vi "Calculate F(x) improved performance.vi"() -> (2 "val1":dbl, 3 "f(x)":dbl)   [LabVIEW 2020]
panel:
  out "Waveform Graph 2":dbl[](graph)
  out "Waveform Graph":dbl[](graph)
  out "Output Array":dbl[][](array[numeric])
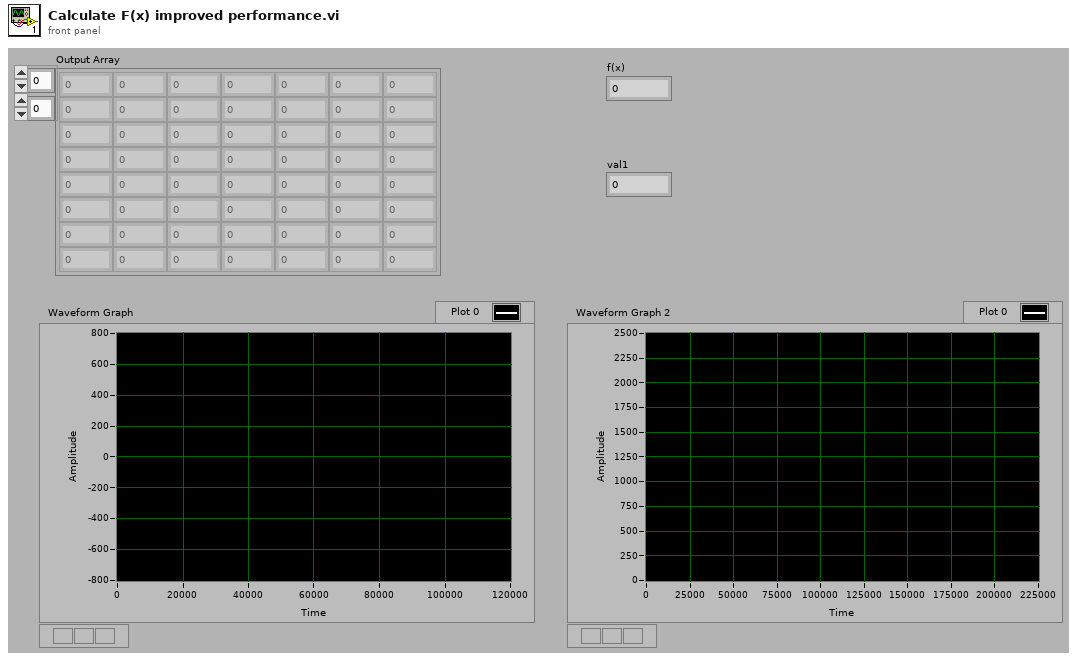
[diagram p1: front panel]
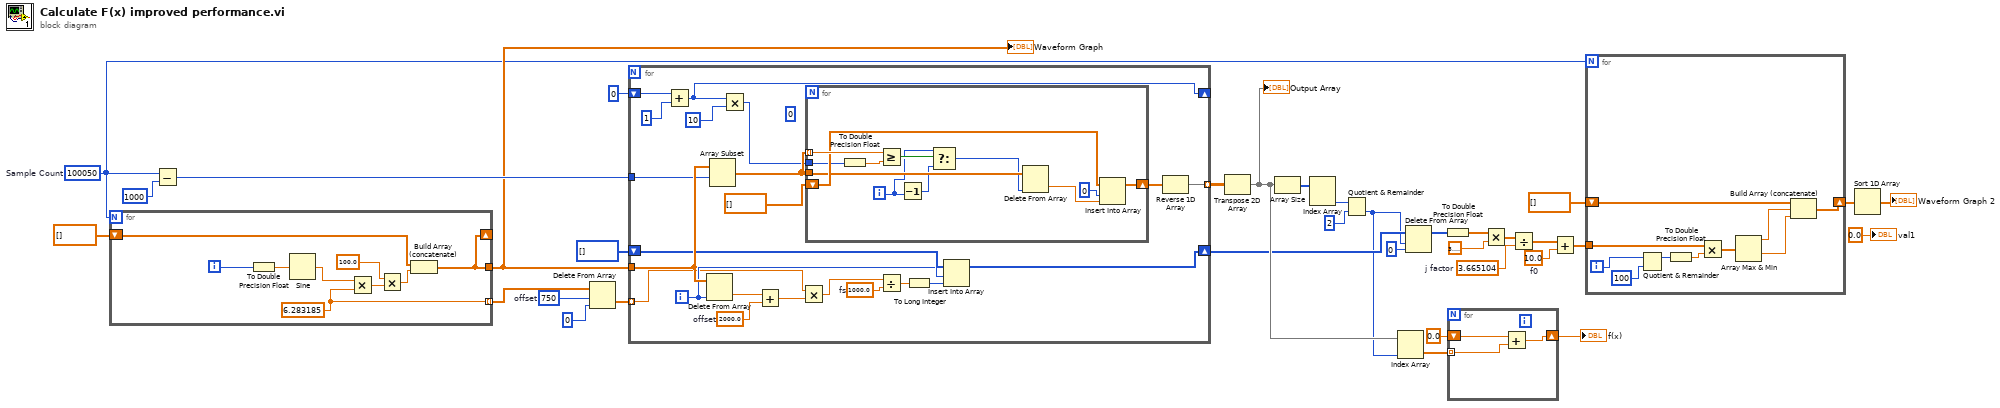
[diagram p0: block diagram]
diagram:
  w10 = 10.0  # f0
  w9 = 3.665104  # j factor
  w17 = 100050  # Sample Count
  w19 = 750  # offset
  n1 = for {
    N: w17 -> [_]
    tunnel: [w38] -> w31 mode=indexing
    tunnel: [w41] -> w18
    shift-right: [w41] -> _
    shift-left: dbl[] [] -> [w40]
    i -> [w42]
    w38 = 6.283185
    n2 = To Double Precision Float(number=w42) -> (double precision float=w43:dbl)
    n3 = Sine(x=w43) -> (sin(x)=w39:dbl)
    n4 = Multiply(x=w39, y=w38) -> (x*y=w37:dbl)
    n5 = Multiply(x=100.0, y=w37) -> (x*y=w35:dbl)
    n6 = Build Array (concatenate)(w40, w35) -> (w41:dbl[])
  }
  "Waveform Graph" <- w18
  n7 = Subtract(x=w17, y=1000) -> (x-y=w22:i32)
  n8 = Delete From Array(array=w31, length=w19, index=0) -> (deleted portion=w20:dbl[])  [unwired: 1 out]
  n9 = for {
    tunnel: w18 -> [w56]
    tunnel: w22 -> [w48]
    tunnel: [w62] -> w34 mode=indexing
    shift-right: [w59] -> _
    shift-left: 0 -> [w60]
    shift-right: [w54] -> w8
    shift-left: i32[] [] -> [w55]
    tunnel: w20 -> [w52] mode=indexing
    i -> [w53]
    w44 = 1000.0  # fs
    w47 = 2000.0  # offset
    (unwired) 0
    n10 = Add(x=w60, y=1) -> (x+y=w59:i32)
    n11 = Delete From Array(array=w56, index=w53) -> (deleted portion=w51:dbl)  [unwired: 1 in, 1 out]
    n12 = Array Subset(array=w56, index=w48) -> (w65:dbl[])  [unwired: 1 in]
    n13 = Multiply(x=w59, y=10) -> (x*y=w57:i32)
    n14 = Add(x=w51, y=w47) -> (x+y=w46:dbl)
    n15 = Multiply(x=w52, y=w46) -> (x*y=w45:dbl)
    n16 = for {
      tunnel: w65 -> [w77] mode=indexing
      tunnel: w65 -> [w74]
      shift-right: [w75] -> w63
      shift-left: dbl[] [] ("array") -> [w76]
      tunnel: w57 -> [w71]
      i -> [w67]
      n17 = To Double Precision Float(number=w71) -> (double precision float=w70:dbl)
      n18 = Greater Or Equal?(x=w77, y=w70) -> (x >= y?=w69:bool)
      n19 = Decrement(x=w67) -> (x-1=w68:i32)
      n20 = Select(t=w67, s=w69, f=w68) -> (s? t:f=w66:i32)
      n21 = Delete From Array(array=w74, index=w66) -> (deleted portion=w72:dbl)  [unwired: 1 in, 1 out]
      n22 = Insert Into Array(array=w76, index=0, new element=w72) -> (w75:dbl[])
    }
    n23 = Divide(x=w45, y=w44) -> (x/y=w50:dbl)
    n24 = To Long Integer(number=w50) -> (32bit integer=w49:i32)
    n25 = Insert Into Array(array=w55, index=w53, new element=w49) -> (w54:i32[])
    n26 = Reverse 1D Array(array=w63) -> (reversed array=w62:dbl[])
  }
  n27 = Transpose 2D Array(2D array=w34) -> (transposed array=w27:dbl[][])
  "Output Array" <- w27
  n28 = Array Size(array=w27) -> (size(s)=w30:i32[])
  n29 = Index Array(array=w30) -> (element #2=w16:i32)  [unwired: 2 in, 1 out]
  n30 = Quotient & Remainder(x=w16, y=2) -> (floor(x/y)=w7:i32)  [unwired: 1 out]
  n31 = Index Array(array=w27, index (col)=w7) -> (element=w26:dbl[])  [unwired: 1 in]
  n32 = Delete From Array(array=w8, length=w7, index=0) -> (array with subset deleted=w14:i32[])  [unwired: 1 out]
  n33 = To Double Precision Float(number=w14) -> (double precision float=w13:dbl[])
  n34 = for {
    tunnel: w26 -> [w80] mode=indexing
    shift-right: [w78] -> w24
    shift-left: 0.0 ("x") -> [w79]
    n35 = Add(x=w79, y=w80) -> (x+y=w78:dbl)
  }
  "f(x)" <- w24
  n36 = Multiply(x=w13, y=3.141592653589793) -> (x*y=w3:dbl[])
  n37 = Divide(x=w3, y=w9) -> (x/y=w12:dbl[])
  n38 = Add(x=w12, y=w10) -> (x+y=w4:dbl[])
  n39 = for {
    N: w17 -> [_]
    shift-right: [w89] -> w6
    shift-left: dbl[] [] -> [w90]
    tunnel: w4 -> [w83]
    i -> [w84]
    n40 = Quotient & Remainder(x=w84, y=100) -> (x-y*floor(x/y)=w86:i32)  [unwired: 1 out]
    n41 = To Double Precision Float(number=w86) -> (double precision float=w87:dbl)
    n42 = Multiply(x=w83, y=w87) -> (x*y=w88:dbl[])
    n43 = Array Max & Min(array=w88) -> (max value=w82:dbl, min value=w81:dbl)  [unwired: 2 out]
    n44 = Build Array (concatenate)(w90, w82, w81) -> (w89:dbl[])
  }
  n45 = Sort 1D Array(array=w6) -> (sorted array=→"Waveform Graph 2":dbl[])
  "val1" <- 0.0 ("val1")
